vi "DetectChange.vi"(9 "Numeric":dbl) -> (1 "Boolean":bool)   [LabVIEW 2020]
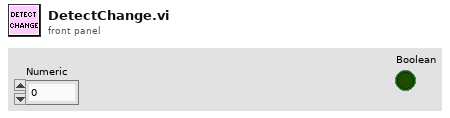
[diagram p1: front panel]
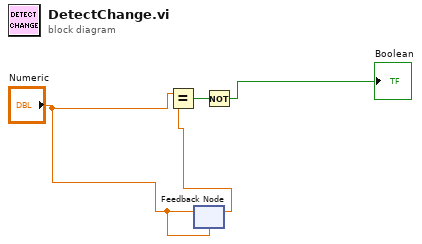
[diagram p0: block diagram]
diagram:
  n1 = feedback #1("Numeric") -> (w4:dbl)
  n2 = Equal?(x="Numeric", y=w4) -> (x = y?=w2:bool)
  n3 = feedback-in #1("Numeric") -> ()
  n4 = Not(x=w2) -> (.not. x?=→"Boolean":bool)
